vi "svx_Continuous Swept-Sine Generator.vi"(4 "chirp settings":T2={"amplitude"=0.0, "frequency range"={"start (Hz)"=20.0, "stop (Hz)"=20000.0, "frequency spacing"=enum."Logarithmic"}, "sampling info"={"Fs"=50000.0, "chirp duration [s]"=3.0}, "initial states"={"frequency [Hz]"=20.0, "phase [rad]"=0.0, "elapsed time [s]"=0.0}, "frequency slope"=0.0, "maximum harmonic"=0, "prefix len [samples]"={"integer"=0, "fractional"=0.0}} {"frequency slope" format="%.2f"; "prefix len [samples]"."fractional" format="%.2p"; "initial states"."elapsed time [s]" format="%.2f"; "initial states"."phase [rad]" format="%.2f"; "initial states"."frequency [Hz]" format="%.2f"; "sampling info"."chirp duration [s]" format="%.2f"; "sampling info"."Fs" format="%.2p"; "frequency range"."stop (Hz)" format="%.2f"; "frequency range"."start (Hz)" format="%.2f"; "amplitude" format="%.2f"}, 5 "signal type":T1(ring), 6 "sampling info":cluster{"Fs":dbl, "#s":dbl}={"Fs"=1000.0, "#s"=1000.0} {"#s" format="%.2p"; "Fs" format="%.2p"}, 7 "generation control":T3(ring), 8 "error in":errorcluster, 9 "delay until transition (0 samples)":i32, 10 "initial waveform state":cluster{"amplitude":dbl, "offset":dbl, "tf":dbl} {"tf" format="%.2f"; "offset" format="%.2f"; "amplitude" format="%.2f"}, 11 "desired waveform state":T4={"amplitude"=1.0, "offset"=0.0, "tf (ignored)"=0.0} {"tf (ignored)" format="%.2f"; "offset" format="%.2p"; "amplitude" format="%.2p"}) -> (0 "error out":errorcluster, 1 "end reached?":bool, 2 "final waveform state":cluster{"amplitude":dbl, "offset":dbl, "tf":dbl} {"tf" format="%.2f"; "offset" format="%.2f"; "amplitude" format="%.2f"}, 3 "signal out":waveform(dbl))   [LabVIEW 2017]
uses:
  <vilib>/addons/_NISVFA/_Generation/subVIs/sv_Chirp Settings.ctl
  <vilib>/addons/_NISVFA/_Generation/SoundVib_Generation.lvlib
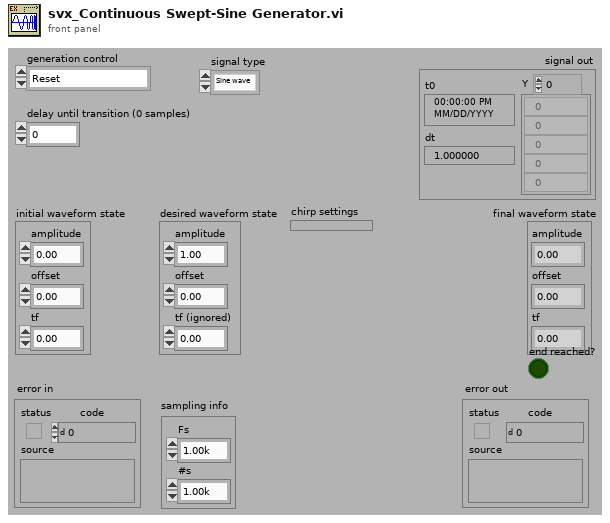
[diagram p1: front panel]
types:
  T1 = enum16{"Sine wave", "Dual tone (IMD)", "Multitone", "Chirp", "Frequency flat chirp", "Uniform white noise", "Gaussian white noise", "Pink noise", "PRN", "Continuous swept-sine"}
  T2 = typedef "SoundVib_Generation.lvlib/sv_Chirp Settings.ctl" = cluster{"amplitude":dbl, "frequency range":cluster{"start (Hz)":dbl, "stop (Hz)":dbl, "frequency spacing":enum16{"Linear", "Logarithmic"}}, "sampling info":cluster{"Fs":dbl, "chirp duration [s]":dbl}, "initial states":cluster{"frequency [Hz]":dbl, "phase [rad]":dbl, "elapsed time [s]":dbl}, "frequency slope":dbl, "maximum harmonic":i32, "prefix len [samples]":cluster{"integer":u32, "fractional":dbl}}
  T3 = enum16{"Reset", "Continue from previous", "Continue from state", "Zero from previous", "Zero from state"}
  T4 = cluster{"amplitude":dbl, "offset":dbl, "tf (ignored)":dbl}
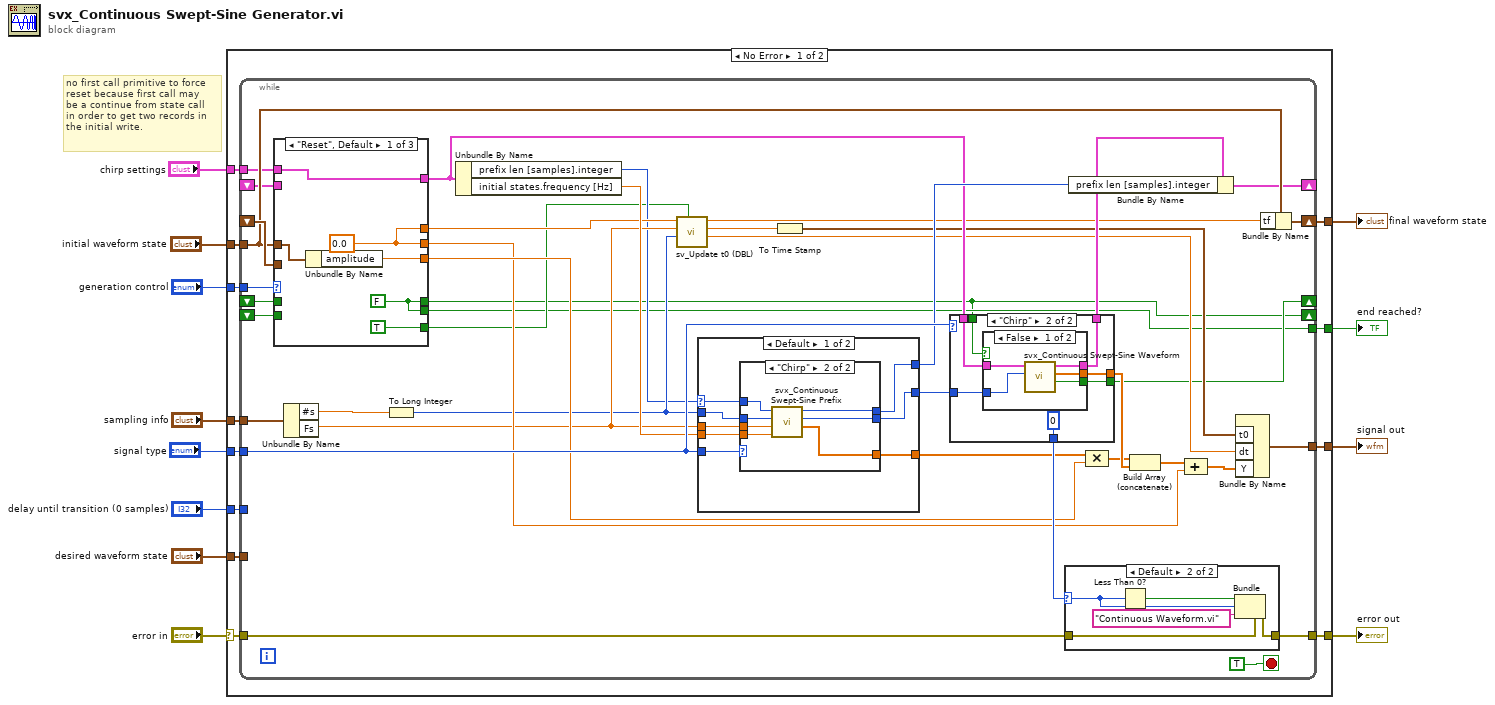
[diagram p0: block diagram]
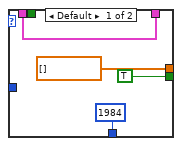
[diagram p2: hidden frame]
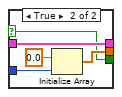
[diagram p3: hidden frame]
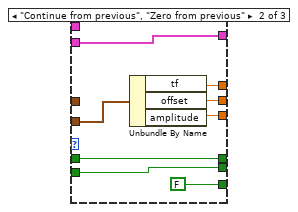
[diagram p5: hidden frame]
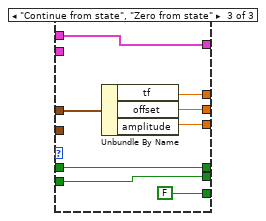
[diagram p6: hidden frame]
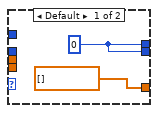
[diagram p7: hidden frame]
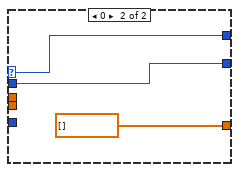
[diagram p8: hidden frame]
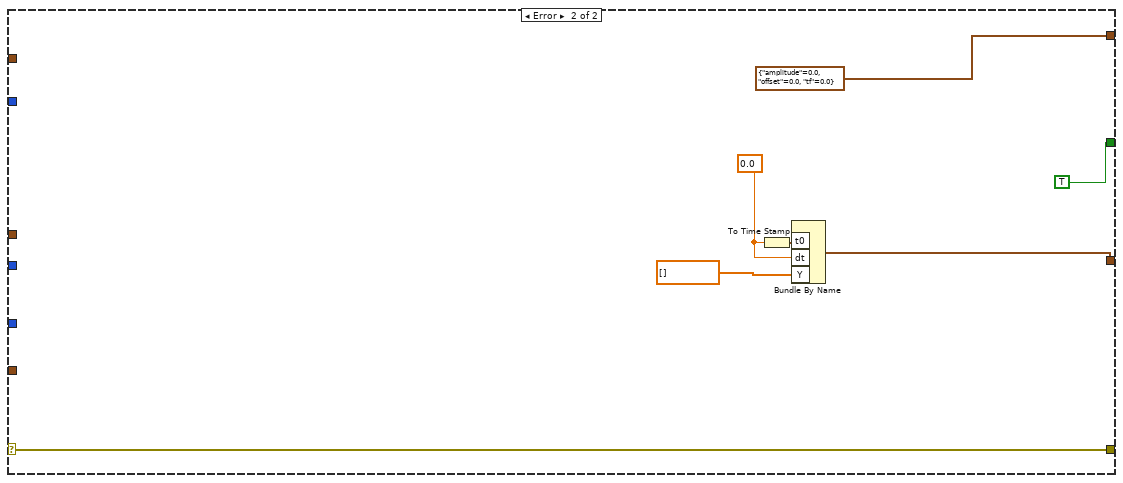
[diagram p9: hidden frame]
diagram:
  # "no first call primitive to force \nreset because first call may \nbe a continue from state call\nin order to get two records in \nthe initial write."
  n1 = case shown="No Error" "error in" {
    selector: "error in" -> [w21 w140]
    tunnel: [w23 w140] -> w11
    tunnel: [w22 w141] -> w4
    tunnel: "delay until transition (0 samples)" -> [w20 _]
    tunnel: [w19 cluster{"amplitude":dbl, "offset":dbl, "tf":dbl} {"amplitude"=0.0, "offset"=0.0, "tf"=0.0} ("initial waveform state")] -> w9
    tunnel: "generation control" -> [w18 _]
    tunnel: "desired waveform state" -> [w17 _]
    tunnel: "initial waveform state" -> [w16 _]
    tunnel: "signal type" -> [w15 _]
    tunnel: "sampling info" -> [w24 _]
    tunnel: "chirp settings" -> [w14 _]
    tunnel: [w13 TRUE ("end reached?")] -> w1
    frame No Error {
      n2 = while {
        tunnel: w16 -> [w60]
        tunnel: w17 -> [_]
        tunnel: w18 -> [w54]
        shift-left: _ -> [w62]
        shift-right: [w57] -> w19
        tunnel: w20 -> [_]
        tunnel: w21 -> [w59]
        tunnel: [w63] -> w22
        tunnel: [w58] -> w23
        tunnel: w15 -> [w53]
        tunnel: w24 -> [w64]
        tunnel: w14 -> [w52]
        shift-right: [w48] -> _
        shift-left: _ -> [w51]
        tunnel: [w26] -> w13
        shift-right: [w28] -> _
        shift-left: _ -> [w32]
        shift-right: [w25] -> _
        shift-left: _ -> [w27]
        stop <- TRUE stop-if-true
        n3 = case shown="\"Reset\", Default" w54 {
          tunnel: w62 -> [_ w105 _]
          tunnel: [TRUE FALSE FALSE] -> w35
          tunnel: [w94 w103 w112] -> w41
          tunnel: [w94 w104 w113] -> w43
          tunnel: w60 -> [w96 _ w111]
          tunnel: [w97 w102 w110] -> w44
          tunnel: w52 -> [w95 _ w109]
          tunnel: [w95 w101 w109] -> w47
          tunnel: w51 -> [_ w101 _]
          tunnel: w32 -> [_ w100 w108]
          tunnel: [w93 w100 w108] -> w25
          tunnel: w27 -> [_ w99 w107]
          tunnel: [w93 w99 w107] -> w26
          frame "Reset", Default {
            w93 = FALSE ("end reached?")
            w94 = 0.0
            n4 = Unbundle By Name(w96) -> ("amplitude"=w97:dbl)
          }
          frame "Continue from previous", "Zero from previous" {
            n5 = Unbundle By Name(w105) -> ("tf"=w103:dbl, "offset"=w104:dbl, "amplitude"=w102:dbl)
          }
          frame "Continue from state", "Zero from state" {
            n6 = Unbundle By Name(w111) -> ("tf"=w112:dbl, "offset"=w113:dbl, "amplitude"=w110:dbl)
          }
        }
        n7 = Unbundle By Name(w64) -> ("#s"=w61:dbl, "Fs"=w40:dbl)
        n8 = To Long Integer(number=w61) -> (32bit integer=w37:i32)
        n9 = Unbundle By Name(w47) -> ("prefix len [samples].integer"=w36:u32, "initial states.frequency [Hz]"=w50:dbl)
        n10 = call <vilib>:"sv_Update t0 (DBL).vi"("Reset Generation"=w35, "samples"=w37, "sample rate (S/s)"=w40, "tf previous"=w41) -> ("dt"=w34:dbl, "t0"=w39:dbl, "tf new"=w38:dbl)  [unwired: 5 in]
        n11 = case shown="Default" w36 {
          selector: w36 -> [w122 w132]
          tunnel: [w115 dbl[] [] ("Sine Wave")] -> w30
          tunnel: [w117 w133] -> w56
          tunnel: w53 -> [w120 _]
          tunnel: w40 -> [w121 _]
          tunnel: w37 -> [w119 w133]
          tunnel: w50 -> [w118 _]
          tunnel: [w116 w132] -> w49
          frame Default {
            n12 = case shown="\"Chirp\"" w120 {
              tunnel: w122 -> [_ w125]
              tunnel: [dbl[] [] ("Periodic Random Noise") w127] -> w115
              tunnel: w121 -> [_ w130]
              tunnel: w119 -> [_ w131]
              tunnel: w118 -> [_ w129]
              tunnel: [w123 w128] -> w116
              tunnel: [w123 w126] -> w117
              frame Default {
                w123 = 0 ("prefix len out [samples]")
              }
              frame "Chirp" {
                n13 = call <vilib>:"svx_Continuous Swept-Sine Prefix.vi"("initial freq [Hz]"=w129, "Fs"=w130, "block size [samples]"=w131, "prefix len [samples]"=w125) -> ("sin(x)"=w127:dbl[], "block size out [samples]"=w126:i32, "prefix len out [samples]"=w128:i32)  [unwired: 5 in]
              }
            }
          }
          frame 0 {
          }
        }
        n14 = To Time Stamp(1:w39) -> (0:w33:timestamp)
        n15 = case shown="\"Chirp\"" w53 {
          tunnel: w56 -> [_ w73]
          tunnel: [dbl[] [] ("Periodic Random Noise") w72] -> w45
          tunnel: [1984 ("error") 0 ("error")] -> w55
          tunnel: w47 -> [w67 w75]
          tunnel: [w67 w74] -> w46
          tunnel: [TRUE ("end reached?") w71] -> w28
          tunnel: w25 -> [_ w70]
          frame Default {
          }
          frame "Chirp" {
            n16 = case shown="False" w70 {
              selector: w70 -> [_ w82]
              tunnel: w75 -> [w81 w86]
              tunnel: [w80 w86] -> w74
              tunnel: w73 -> [w79 w85]
              tunnel: [w78 w83] -> w72
              tunnel: [w77 w82] -> w71
              frame False {
                n17 = call <vilib>:"svx_Continuous Swept-Sine Waveform.vi"("block size [samples]"=w79, "chirp settings"=w81) -> ("end reached?"=w77:bool, "chirp signal"=w78:dbl[], "chirp settings out"=w80:T2)  [unwired: 7 in]
              }
              frame True {
                n18 = Initialize Array(0.0 ("element"), w85) -> (w83:dbl[])
              }
            }
          }
        }
        n19 = case shown="Default" w55 {
          selector: w55 -> [_ w91]
          tunnel: w59 -> [w87 w92]
          tunnel: [w87 w88] -> w58
          frame 0 {
          }
          frame Default {
            n20 = Less Than 0?(x=w91) -> (x < 0?=w90:bool)
            n21 = Bundle(cluster=w92, "status"=w90, "code"=w91, "source"="Continuous Waveform.vi" ("subVI Name")) -> (w88:errorcluster)
          }
        }
        n22 = Bundle By Name(cluster=w46, "prefix len [samples].integer"=w49) -> (w48:T2)
        n23 = Compound Arithmetic op=MULTIPLY(w30, w44) -> (w31:dbl[])
        n24 = Build Array (concatenate)(w31, w45) -> (w29:dbl[])
        n25 = Compound Arithmetic op=ADD(w29, w43) -> (w42:dbl[])
        n26 = Bundle By Name("t0"=w33, "dt"=w34, "Y"=w42) -> (w63:waveform(dbl))  [unwired: 1 in]
        n27 = Bundle By Name(cluster=w60, "tf"=w38) -> (w57:cluster{"amplitude":dbl, "offset":dbl, "tf":dbl})
      }
    }
    frame Error {
      w138 = 0.0 ("t0")
      n28 = To Time Stamp(1:w138) -> (0:w136:timestamp)
      n29 = Bundle By Name("t0"=w136, "dt"=w138, "Y"=dbl[] []) -> (w141:waveform(dbl))  [unwired: 1 in]
    }
  }
  "error out" <- w11
  "signal out" <- w4
  "final waveform state" <- w9
  "end reached?" <- w1
